vi "Calculate Tension.vi"(8 "t < X ?":bool, 9 "Wire Length":dbl, 10 "Linear Density":dbl, 11 "Frequency":dbl) -> (1 "Linear Density":dbl, 2 "Wire Length":dbl, 3 "Tension":dbl)   [LabVIEW 2018]
panel:
  # "Inputs"
  # "Outputs"
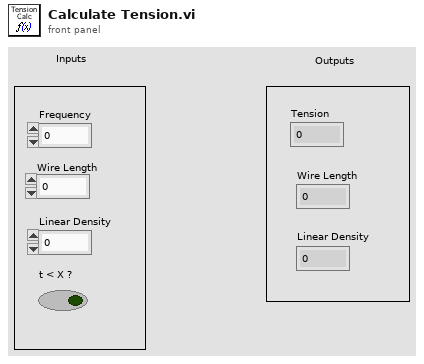
[diagram p1: front panel]
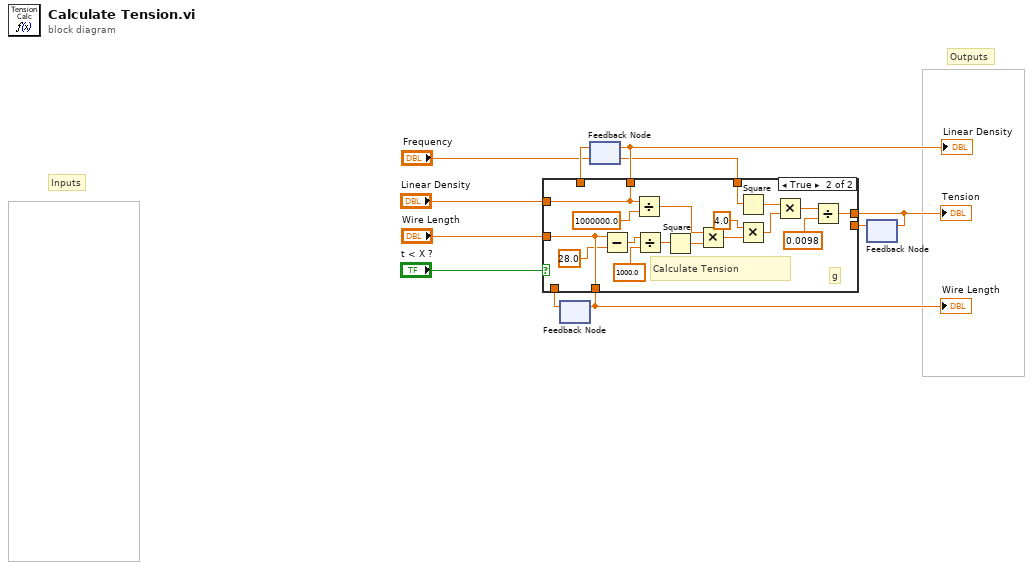
[diagram p0: block diagram]
diagram:
  # "Outputs"
  # "Inputs"
  n1 = feedback #1() -> (w7:dbl)  [unwired: 1 in]
  n2 = feedback #2() -> (w5:dbl)  [unwired: 1 in]
  n3 = feedback #3() -> (w9:dbl)  [unwired: 1 in]
  n4 = case shown="True" "t < X ?" {
    tunnel: "Frequency" -> [_ w19]
    tunnel: [w13 w28] -> w10
    tunnel: w9 -> [w13 _]
    tunnel: "Linear Density" -> [_ w22]
    tunnel: "Wire Length" -> [_ w16]
    tunnel: [w11 w16] -> w8
    tunnel: w7 -> [w11 _]
    tunnel: [w12 w22] -> w6
    tunnel: w5 -> [w12 _]
    frame False {
    }
    frame True {
      # "g"
      # "Calculate Tension"
      n5 = Subtract(x=w16, y=28.0) -> (x-y=w15:dbl)
      n6 = Divide(x=w22, y=1000000.0) -> (x/y=w29:dbl)
      n7 = Divide(x=w15, y=1000.0) -> (x/y=w18:dbl)
      n8 = Square(x=w18) -> (x^2=w17:dbl)
      n9 = Multiply(x=w29, y=w17) -> (x*y=w25:dbl)
      n10 = Square(x=w19) -> (x^2=w20:dbl)
      n11 = Multiply(x=4.0, y=w25) -> (x*y=w30:dbl)
      n12 = Multiply(x=w20, y=w30) -> (x*y=w27:dbl)
      n13 = Divide(x=w27, y=0.0098) -> (x/y=w28:dbl)
    }
  }
  "Tension" <- w10
  "Wire Length" <- w8
  "Linear Density" <- w6
  n14 = feedback-in #1(w8) -> ()
  n15 = feedback-in #2(w6) -> ()
  n16 = feedback-in #3(w10) -> ()
